vi "FindClosestOrientation.vi"(8 "wheel":T1(ring), 10 "desired angle (radians)":dbl, 11 "desired speed":dbl) -> (0 "current angle (radians)":dbl, 1 "reversed?":bool, 2 "closest angle (radians)":dbl, 3 "closest speed":dbl)   [LabVIEW 2013]
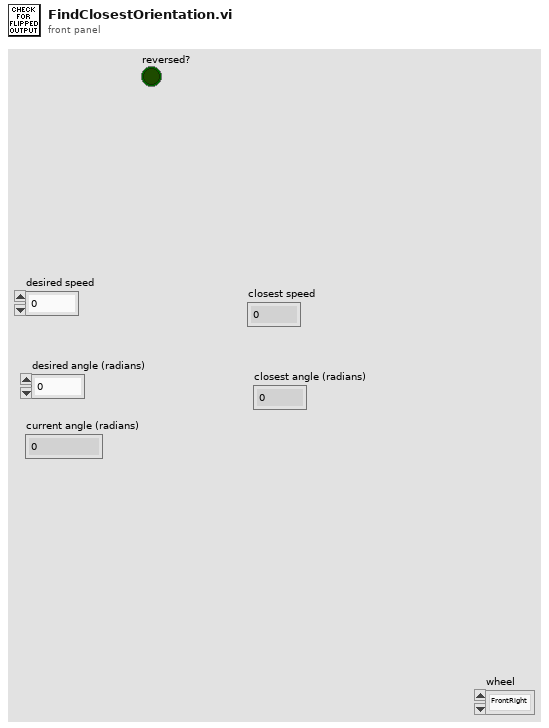
[diagram p1: front panel]
types:
  T1 = enum16{"FrontRight", "FrontLeft", "RearRight", "RearLeft", ""}
  T2 = typedef "WPI_EncoderDevRef.ctl" = cluster{"DevStatus":errorcluster, "EncoderIndex":T3, "CounterIndex":T4, "DistancePerCount":dbl, "Decoding Type":T5}
  T3 = typedef "FPGA_EncoderIdx.ctl" = enum8{"Enc 0", "Enc 1", "Enc 2", "Enc 3", "Invalid"}
  T4 = typedef "FPGA_CounterCtrSystemIndex.ctl" = enum8{"Ctr 0", "Ctr 1", "Ctr 2", "Ctr 3", "Ctr 4", "Ctr 5", "Ctr 6", "Ctr 7", "Invalid"}
  T5 = typedef "WPI_EncoderType.ctl" = enum16{"1x", "2x", "4x"}
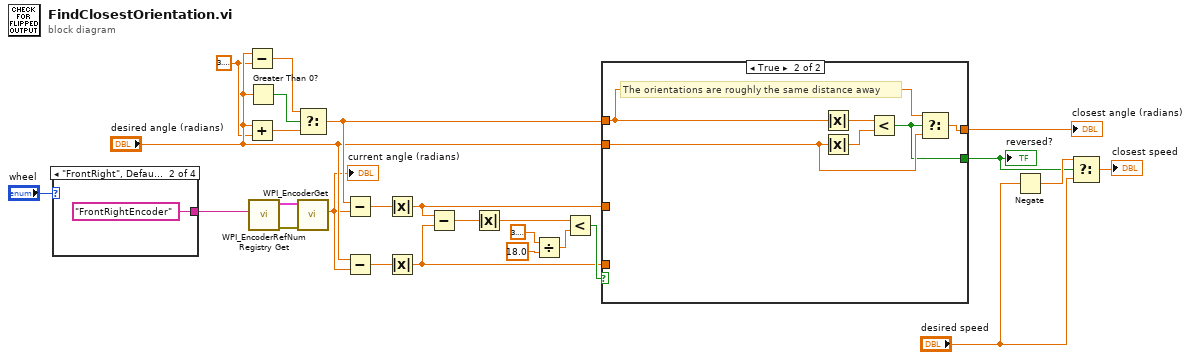
[diagram p0: block diagram]
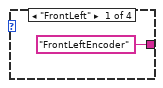
[diagram p2: hidden frame]
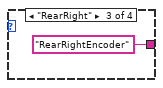
[diagram p3: hidden frame]
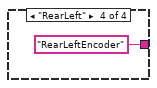
[diagram p4: hidden frame]
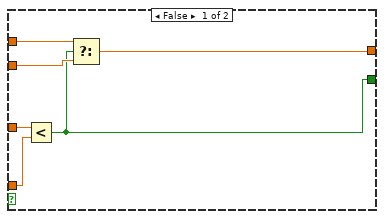
[diagram p5: hidden frame]
diagram:
  w4 = 3.141592653589793
  n1 = case shown="\"FrontRight\", Default" "wheel" {
    tunnel: ["FrontLeftEncoder" "FrontRightEncoder" "RearRightEncoder" "RearLeftEncoder"] -> w5
    frame "FrontLeft" {
    }
    frame "FrontRight", Default {
    }
    frame "RearRight" {
    }
    frame "RearLeft" {
    }
  }
  n2 = Subtract(x="desired angle (radians)", y=w4) -> (x-y=w24:dbl)
  n3 = Add(x="desired angle (radians)", y=w4) -> (x+y=w25:dbl)
  n4 = Greater Than 0?(x="desired angle (radians)") -> (x > 0?=w26:bool)
  n5 = call <vilib>:"WPI_EncoderRefNum Registry Get.vi"("refnum name"=w5) -> ("error out"=w6:errorcluster, "EncoderDevRef"=w7:T2)  [unwired: 9 in]
  n6 = Select(t=w24, s=w26, f=w25) -> (s? t:f=w18:dbl)
  n7 = call <vilib>:"WPI_EncoderGet.vi"("error in (no error)"=w6, "EncoderDevRef"=w7) -> ("Distance"=w9:dbl)  [unwired: 4 in, 5 out]
  "current angle (radians)" <- w9
  n8 = Subtract(x=w18, y=w9) -> (x-y=w23:dbl)
  n9 = Subtract(x="desired angle (radians)", y=w9) -> (x-y=w22:dbl)
  n10 = Absolute Value(x=w23) -> (abs(x)=w16:dbl)
  n11 = Absolute Value(x=w22) -> (abs(x)=w15:dbl)
  n12 = Subtract(x=w16, y=w15) -> (x-y=w21:dbl)
  n13 = Absolute Value(x=w21) -> (abs(x)=w20:dbl)
  n14 = Divide(x=3.141592653589793, y=18.0) -> (x/y=w1:dbl)
  n15 = Less?(x=w20, y=w1) -> (x < y?=w19:bool)
  n16 = case shown="True" w19 {
    tunnel: w18 -> [w34 w40]
    tunnel: "desired angle (radians)" -> [w33 w39]
    tunnel: [w32 w38] -> w14
    tunnel: w16 -> [w36 _]
    tunnel: w15 -> [w35 _]
    tunnel: [w31 w37] -> w12
    frame False {
      n17 = Less?(x=w36, y=w35) -> (x < y?=w31:bool)
      n18 = Select(t=w34, s=w31, f=w33) -> (s? t:f=w32:dbl)
    }
    frame True {
      # "The orientations are roughly the same distance away"
      n19 = Absolute Value(x=w40) -> (abs(x)=w42:dbl)
      n20 = Absolute Value(x=w39) -> (abs(x)=w41:dbl)
      n21 = Less?(x=w42, y=w41) -> (x < y?=w37:bool)
      n22 = Select(t=w40, s=w37, f=w39) -> (s? t:f=w38:dbl)
    }
  }
  "reversed?" <- w12
  "closest angle (radians)" <- w14
  n23 = Negate(x="desired speed") -> (-x=w13:dbl)
  n24 = Select(t=w13, s=w12, f="desired speed") -> (s? t:f=→"closest speed":dbl)
